vi "Excel___Write System Information.vi"() -> ()   [LabVIEW 2013]
panel:
  out "# of Standards":i32
  out "Error Out":errorcluster
  out "Sheets Ref Out":refnum<k7>
  in  "Error In":errorcluster
  in  "Sheets Ref In":refnum<k7>
  in  "Cal Cert Started":bool
  in  "Cal Certificate Path":path
  in  "Cal Cert Template Path":path
  in  "Calibration Details":string[][](table)=[["Calibrator Name", "Procedure", "Calibration Interval", "Date Complete", "Date Due", "Calibrator Signature"]]
  in  "Instrument Identification":string[][](table)=[["Gauge Number:"], ["Common Identifier:"], ["Manufacturer:"], ["Model Number:"], ["Description:"], ["Serial Number:"], ["In-Service Date:"], ["Condition:"]]
  in  "Environment Details":string[][](table)=[["Company:", "TI Automotive"], ["Building:", "Caro Test Center"], ["Street Address:", "628 Columbia St."], ["City Address:", "Caro, MI 48723"], ["Room Name:", ""], ["Room Temperature:", ""], ["Room Humidity:", ""]]
  in  "Standards Used":string[][](table)=[["Description:", "Gauge Number:", "Units:", "Unit Abbreviation:", "Calibration Due:"]]
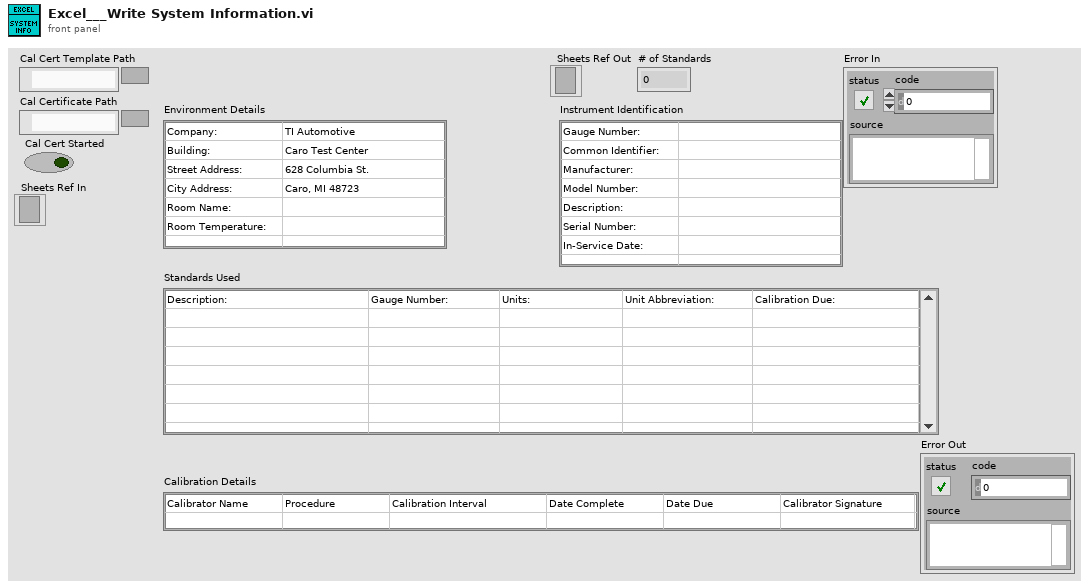
[diagram p1: front panel]
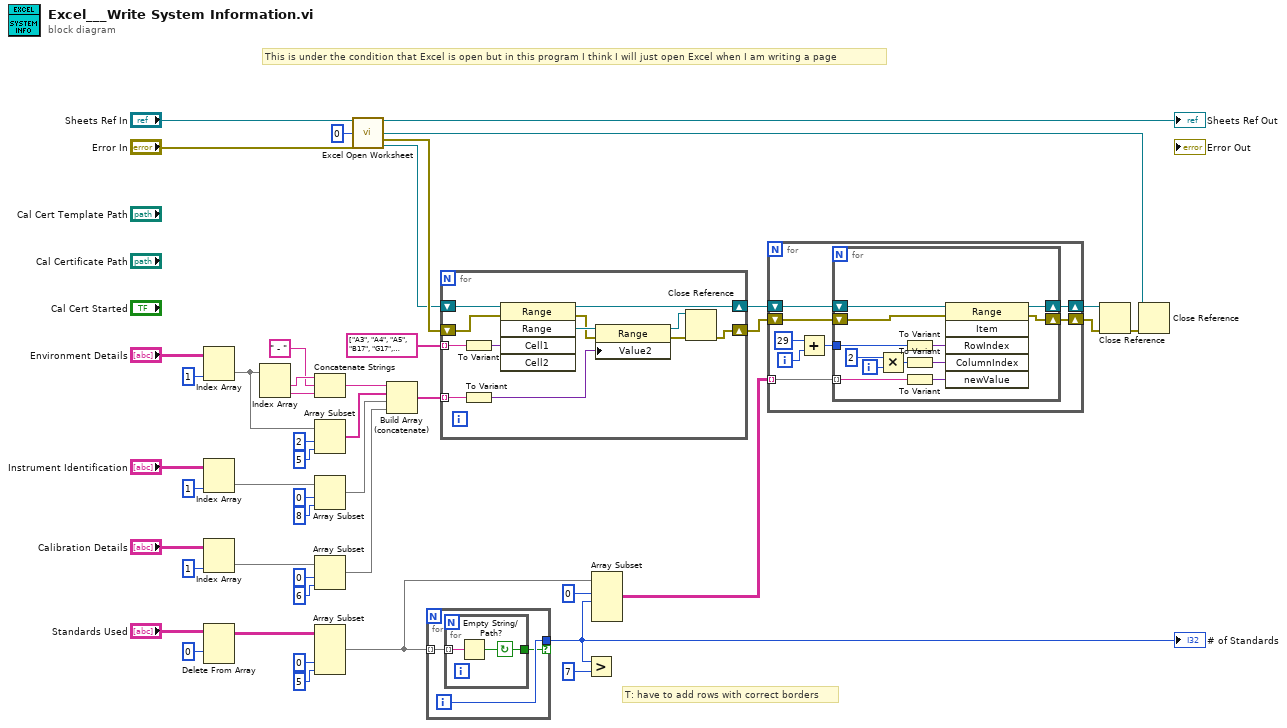
[diagram p0: block diagram]
diagram:
  # "T: have to add rows with correct borders"
  # "This is under the condition that Excel is open but in this program I think I will just open Excel when I am writing a page"
  n1 = Index Array(array="Environment Details", index (col)=1 ("disabled index (col)")) -> (element=w34:string[])  [unwired: 1 in]
  n2 = Index Array(array="Instrument Identification", index (col)=1 ("disabled index (col)")) -> (element=w31:string[])  [unwired: 1 in]
  n3 = Index Array(array="Calibration Details", index (col)=1 ("disabled index (col)")) -> (element=w26:string[])  [unwired: 1 in]
  n4 = Delete From Array(array="Standards Used", index (row)=0) -> (array with subset deleted=w11:string[][])  [unwired: 2 in, 1 out]
  n5 = Index Array(array=w34) -> (element #1=w43:string, element #2=w42:string)  [unwired: 2 in]
  n6 = Concatenate Strings(w43, " - ", w42) -> (w25:string)
  n7 = Array Subset(array=w34, index=2, length=5) -> (w24:string[])
  n8 = Array Subset(array=w31, index=0, length=8) -> (w23:string[])
  n9 = Array Subset(array=w26, index=0, length=6) -> (w22:string[])
  n10 = Array Subset(array=w11, index (col)=0 ("index"), length (col)=5 ("length")) -> (w7:string[][])  [unwired: 2 in]
  n11 = call "Excel Open Worksheet.vi"("Sheets Ref In"="Sheets Ref In", "Sheet#"=0, "Error In"="Error In") -> ("Sheets Ref Out"=→"Sheets Ref Out":refnum<k7>, "Worksheet Ref Out"=w13:refnum<k7>, "Error Out"=w15:errorcluster, "Cells Ref Out"=w14:refnum<k7>)  [unwired: 9 in]
  n12 = Build Array (concatenate)(w25, w24, w23, w22) -> (w17:string[])
  n13 = for {
    tunnel: w7 -> [w48] mode=indexing
    tunnel: [w47] -> w5 if=w46
    i -> [w47]
    n14 = for {
      tunnel: w48 -> [w50] mode=indexing
      tunnel: [w49] -> w46
      stop <- w49 continue-if-true
      n15 = Empty String/Path?(string/path=w50) -> (empty?=w49:bool)
    }
  }
  "# of Standards" <- w5
  n16 = for {
    shift-right: [w57] -> w3
    shift-left: w15 -> [w62]
    shift-right: [w56] -> w4
    shift-left: w14 -> [w55]
    tunnel: w17 -> [w54] mode=indexing
    tunnel: string[] ["A3", "A4", "A5", "B17", "G17", "G19", "B8", "G8", "B10", "B12", "G10", "B14", "G12", "G14", "B22", "G22", "B24", "B26", "G24", "G26"] -> [w53] mode=indexing
    n17 = To Variant(anything=w53) -> (Variant=w60:variant)
    n18 = To Variant(anything=w54) -> (Variant=w58:variant)
    n19 = invoke class="Range" method="Range"(reference=w55, error in=w62, "Cell1"=w60) -> (reference out=w56:refnum<k7>, error out=w59:errorcluster, "Range"=w61:refnum<k7>)  [unwired: 2 in, 2 out]
    n20 = property class="Range"(reference=w61, error in=w59, "Value2"=w58) -> (reference out=w52:refnum<k7>, error out=w51:errorcluster)
    n21 = Close Reference(reference=w52, error in (no error)=w51) -> (error out=w57:errorcluster)
  }
  n22 = Greater?(x=w5, y=7) -> ()  [unwired: 1 out]
  n23 = Array Subset(array=w7, index (row)=0 ("index"), length (row)=w5) -> (w2:string[][])  [unwired: 2 in]
  n24 = for {
    shift-right: [w68] -> _
    shift-left: w4 -> [w70]
    shift-right: [w67] -> w1
    shift-left: w3 -> [w69]
    tunnel: w2 -> [w66] mode=indexing
    i -> [w65]
    n25 = Add(x=29, y=w65) -> (x+y=w63:i32)
    n26 = for {
      shift-right: [w80] -> w68
      shift-left: w70 -> [w82]
      shift-right: [w77] -> w67
      shift-left: w69 -> [w81]
      tunnel: w66 -> [w79] mode=indexing
      tunnel: w63 -> [w74]
      i -> [w73]
      n27 = Multiply(x=2, y=w73) -> (x*y=w71:i32)
      n28 = To Variant(anything=w74) -> (Variant=w76:variant)
      n29 = To Variant(anything=w71) -> (Variant=w75:variant)
      n30 = To Variant(anything=w79) -> (Variant=w78:variant)
      n31 = invoke class="Range" method="Item"(reference=w82, error in=w81, "RowIndex"=w76, "ColumnIndex"=w75, "newValue"=w78) -> (reference out=w80:refnum<k7>, error out=w77:errorcluster)  [unwired: 1 in, 4 out]
    }
  }
  n32 = Close Reference(reference=w4, error in (no error)=w1) -> (error out=w18:errorcluster)
  n33 = Close Reference(reference=w13, error in (no error)=w18) -> ()  [unwired: 1 out]
